vi "Post Step Write Single Register.vi"(10 "Write Register Step Data":T1, 11 "Sequence Context In":refnum<k7>) -> (0 "error out":errorcluster, 1 "Set Data":i32[](array[numeric]), 2 "starting address":u16[](array[numeric]) format="%x", 3 "Report Text":string, 4 "Slave unit IDs":u8[](array[numeric]))   [LabVIEW 2023, in "LTT_TeststandSteptypes.lvlib"]
uses:
  LTT_TeststandSteptypes.lvlib
  Control/Write Control.ctl
  HardwareAbstractionLayer_LVOOP/Modbus/Modbus_class/Teststand Steptypes/Control/Modubs FGV State.ctl
  HardwareAbstractionLayer_LVOOP/Modbus/Modbus_class/Modbus.lvclass
  HardwareAbstractionLayer_LVOOP/Database/Database.lvclass
  HardwareAbstractionLayer_LVOOP/Database/SQL Public VI/Control/DB Options.ctl
panel:
  in  "Modbus RTU":T2={"unit ID"=1, "serial type"=enum."RTU", "baud rate"=9600, "parity (even)"=2, "flow control (none)"=0, "VISA resource name"=""} {"flow control (none)" items=["None", "XON/XOFF", "RTS/CTS", "XON/XOFF & RTS/CTS", "DTR/DSR", "XON/XOFF & DTR/DSR"]; "parity (even)" items=["None", "Odd", "Even", "Mark", "Space"]}
  in  "error in":errorcluster
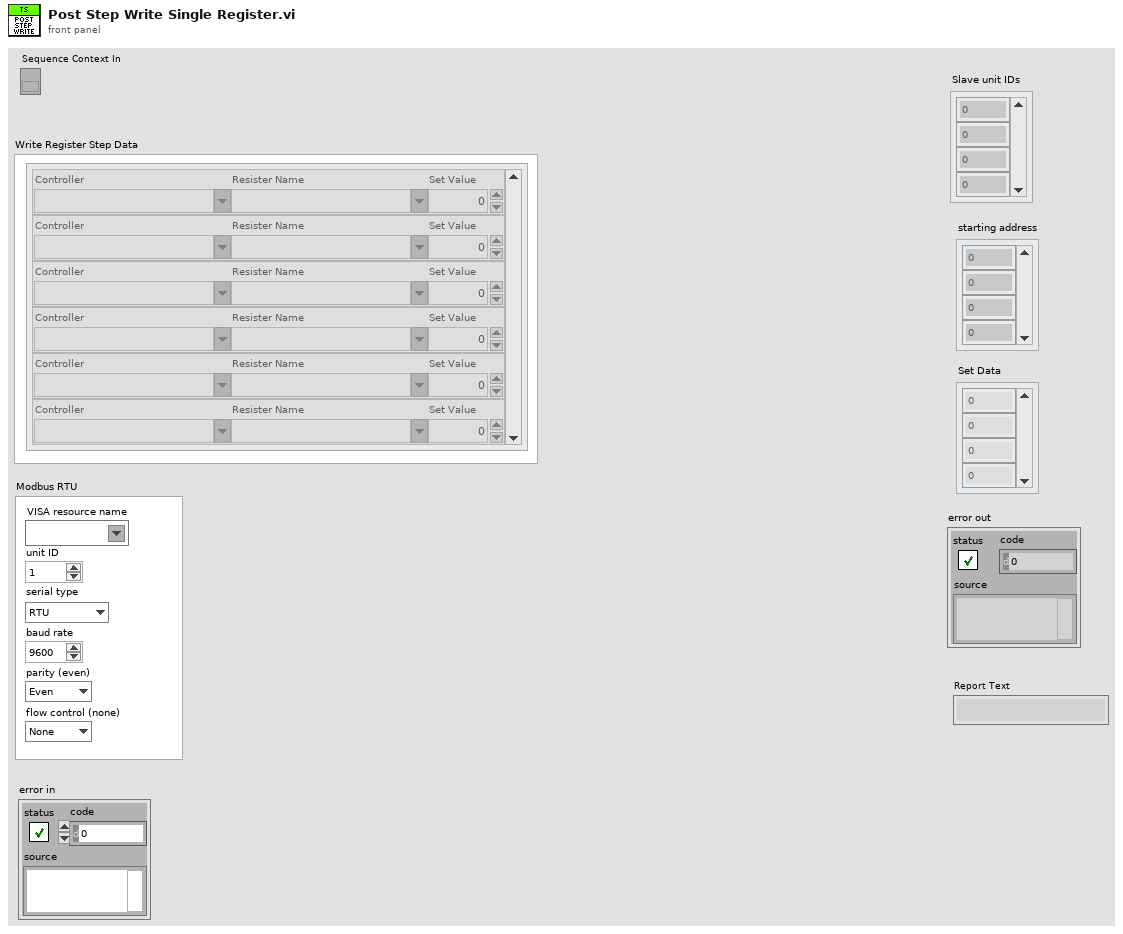
[diagram p1: front panel]
types:
  T1 = typedef "LTT_TeststandSteptypes.lvlib/Write Control.ctl" = cluster{"Edit Controller":cluster{"Controller":string, "Resister Name":string, "Set Value":i32}[]}
  T2 = cluster{"unit ID":u8, "serial type":enum16{"RTU", "ASCII"}, "baud rate":u32, "parity (even)":u16, "flow control (none)":u16, "VISA resource name":refnum<visa-resource-name>}
  T3 = typedef "HardwareAbstractionLayer_LVOOP.lvlib/Database.lvclass/DB Options.ctl" = enum16{"Init", "Select Data", "Insert Data", "Update Data", "Delete Data", "Execute Query", "Create Schema", "Create Table", "List Tables", "List Columns", "Close"}
  T4 = typedef "HardwareAbstractionLayer_LVOOP.lvlib/Modbus.lvclass/Modubs FGV State.ctl" = enum16{"Set", "Get"}
  T5 = cluster{"Controller":string, "Resister Name":string, "Set Value":i32}[]
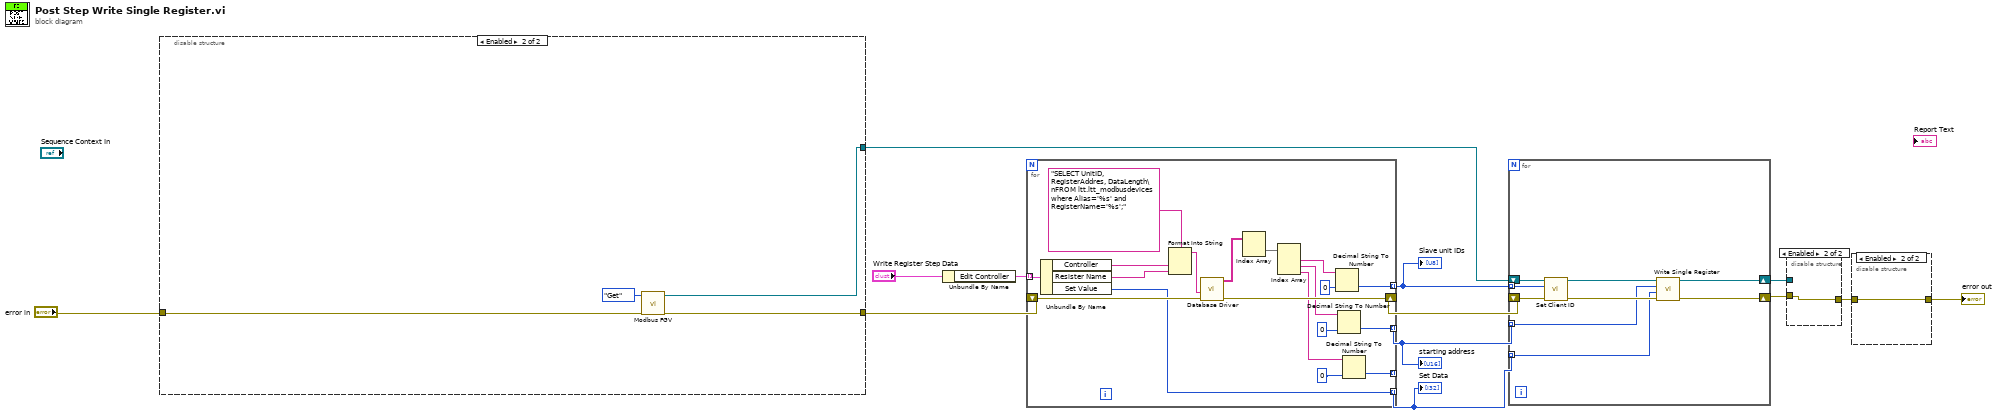
[diagram p0: block diagram]
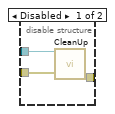
[diagram p2: hidden frame]
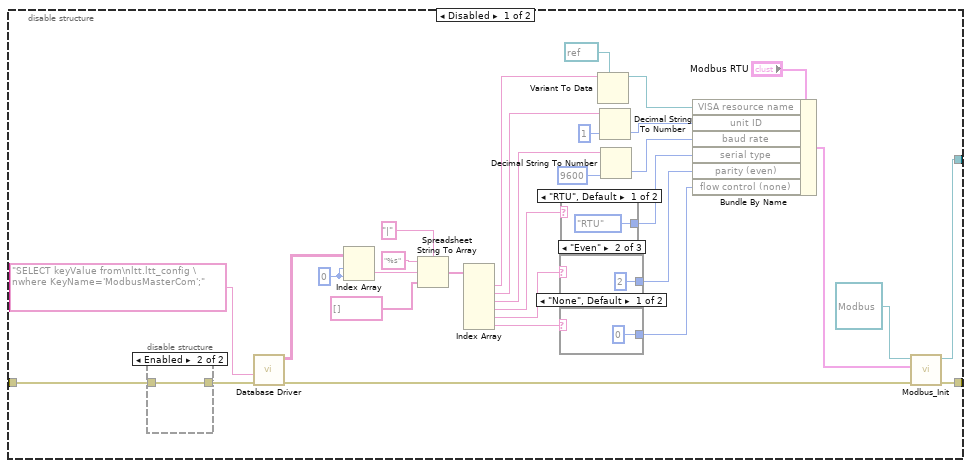
[diagram p3: hidden frame]
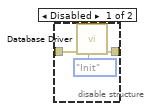
[diagram p4: hidden frame]
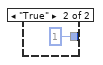
[diagram p5: hidden frame]
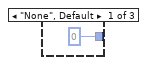
[diagram p6: hidden frame]
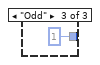
[diagram p7: hidden frame]
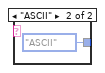
[diagram p8: hidden frame]
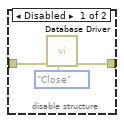
[diagram p9: hidden frame]
diagram:
  n1 = disable-structure shown="Enabled" {
    disable-tunnel: "error in" -> [w43 w59]
    disable-tunnel: [w15 w58] -> w8
    disable-tunnel: [w14 w57] -> w6
    frame Disabled {
      w38 = 0 ("index (row)")
      n2 = disable-structure shown="Enabled" {
        disable-tunnel: w43 -> [w46 w48]
        disable-tunnel: [w45 w48] -> w42
        frame Disabled {
          n3 = call "Database Driver.vi"("Options"=DB_Options."Init", "error in"=w46) -> ("error out"=w45:errorcluster)  [unwired: 6 in, 3 out]
        }
        frame Enabled {
        }
      }
      n4 = call "Database Driver.vi"("error in"=w42, "SQL query"="SELECT keyValue from\nltt.ltt_config \nwhere KeyName='ModbusMasterCom';") -> ("error out"=w41:errorcluster, "data"=w39:string[][])  [unwired: 6 in, 2 out]
      n5 = Index Array(array=w39, index (row)=w38, index (col)=w38) -> (element=w37:string)
      n6 = Spreadsheet String To Array(delimiter (Tab)="|" ("format string"), format string="%s", spreadsheet string=w37, array type (2D Dbl)=string[] []) -> (array=w35:string[])
      n7 = Index Array(array=w35) -> (element #1=w19:string, element #2=w32:string, element #3=w29:string, element #4=w26:string, element #5=w24:string, element #6=w23:string)  [unwired: 6 in]
      n8 = case shown="\"Even\"" w24 {
        tunnel: [u16 0 ("parity (even)") u16 2 ("parity (even)") u16 1 ("parity (even)")] -> w22
        frame "None", Default {
        }
        frame "Even" {
        }
        frame "Odd" {
        }
      }
      n9 = case shown="\"None\", Default" w23 {
        tunnel: [u16 0 ("flow control (none)") u16 1 ("flow control (none)")] -> w21
        frame "None", Default {
        }
        frame "True" {
        }
      }
      n10 = case shown="\"RTU\", Default" w26 {
        tunnel: [enum16{"RTU", "ASCII"}."RTU" ("serial type") enum16{"RTU", "ASCII"}."ASCII" ("serial type")] -> w25
        frame "RTU", Default {
        }
        frame "ASCII" {
        }
      }
      n11 = Variant To Data(type=refnum<visa-resource-name> refnum ("VISA resource name"), Variant=w19) -> (data=w18:refnum<visa-resource-name>)  [unwired: 1 in, 1 out]
      n12 = Decimal String To Number(string=w32, default (0L)=u8 1 ("unit ID")) -> (number=w30:u8)  [unwired: 1 in, 1 out]
      n13 = Decimal String To Number(string=w29, default (0L)=u32 9600 ("baud rate")) -> (number=w28:u32)  [unwired: 1 in, 1 out]
      n14 = Bundle By Name(cluster="Modbus RTU", "VISA resource name"=w18, "unit ID"=w30, "baud rate"=w28, "serial type"=w25, "parity (even)"=w22, "flow control (none)"=w21) -> (w33:T2)
      n15 = call "Modbus_Init.vi"("error in (no error)"=w41, "Modbus RTU"=w33, "object in"=refnum<class "Modbus.lvclass"> refnum ("VT_LTT.lvlib:Modbus")) -> ("error out"=w15:errorcluster, "object out"=w14:refnum<class "Modbus.lvclass">)  [unwired: 7 in]
    }
    frame Enabled {
      n16 = call "Modbus FGV.vi"("error in"=w59, "Action"=Modubs_FGV_State."Get") -> ("error out"=w58:errorcluster, "Modbus Ref"=w57:refnum<class "Modbus.lvclass">)  [unwired: 8 in]
    }
  }
  n17 = Unbundle By Name("Write Register Step Data") -> ("Edit Controller"=w2:T5)
  n18 = for {
    shift-right: [w77] -> w7
    shift-left: w8 -> [w78]
    tunnel: w2 -> [w74] mode=indexing
    tunnel: [w67] -> w5 mode=indexing
    tunnel: [w64] -> w4 mode=indexing
    tunnel: [w61] -> _ mode=indexing
    tunnel: [w60] -> w1 mode=indexing
    n19 = Unbundle By Name(w74) -> ("Controller"=w73:string, "Resister Name"=w72:string, "Set Value"=w60:i32)
    n20 = Format Into String(format string="SELECT UnitID, RegisterAddres, DataLength\nFROM ltt.ltt_modbusdevices where Alias='%s' and RegisterName='%s';", w73, w72) -> (resulting string=w75:string)  [unwired: 2 in, 1 out]
    n21 = call "Database Driver.vi"("error in"=w78, "SQL query"=w75) -> ("error out"=w77:errorcluster, "data"=w71:string[][])  [unwired: 6 in, 2 out]
    n22 = Index Array(array=w71) -> (element=w70:string[])  [unwired: 2 in]
    n23 = Index Array(array=w70) -> (element #1=w69:string, element #2=w65:string, element #3=w63:string)  [unwired: 3 in]
    n24 = Decimal String To Number(string=w69, default (0L)=u8 0 ("Slave unit ID")) -> (number=w67:u8)  [unwired: 1 in, 1 out]
    n25 = Decimal String To Number(string=w65, default (0L)=u16 0 ("starting address")) -> (number=w64:u16)  [unwired: 1 in, 1 out]
    n26 = Decimal String To Number(string=w63, default (0L)=u16 0 ("number of inputs")) -> (number=w61:u16)  [unwired: 1 in, 1 out]
  }
  "Slave unit IDs" <- w5
  "starting address" <- w4
  "Set Data" <- w1
  n27 = for {
    shift-right: [w82] -> w13
    shift-left: w6 -> [w87]
    shift-right: [w84] -> w12
    shift-left: w7 -> [w86]
    tunnel: w5 -> [w81] mode=indexing
    tunnel: w4 -> [w80] mode=indexing
    tunnel: w1 -> [w79] mode=indexing
    n28 = call-dynamic "Set Client ID.vi"("error in (no error)"=w86, "Slave unit ID"=w81, "Modbus in"=w87) -> ("error out"=w85:errorcluster, "Modbus out"=w83:refnum<class "Modbus.lvclass">)  [unwired: 7 in]
    n29 = call-dynamic "Write Single Register.vi"("error in (no error)"=w85, "Write Value"=w79, "Write address"=w80, "Modbus in"=w83) -> ("error out"=w84:errorcluster, "Modbus out"=w82:refnum<class "Modbus.lvclass">)  [unwired: 6 in]
  }
  n30 = disable-structure shown="Enabled" {
    disable-tunnel: w13 -> [w90 _]
    disable-tunnel: w12 -> [w89 w91]
    disable-tunnel: [w88 w91] -> w10
    frame Disabled {
      n31 = call-dynamic "CleanUp.vi"("object in"=w90, "error in (no error)"=w89) -> ("error out"=w88:errorcluster)  [unwired: 16 in, 1 out]
    }
    frame Enabled {
    }
  }
  n32 = disable-structure shown="Enabled" {
    disable-tunnel: w10 -> [w94 w95]
    disable-tunnel: [w93 w95] -> w9
    frame Disabled {
      n33 = call "Database Driver.vi"("Options"=DB_Options."Close", "error in"=w94) -> ("error out"=w93:errorcluster)  [unwired: 6 in, 3 out]
    }
    frame Enabled {
    }
  }
  "error out" <- w9
